vi "RxImgWithCLUT.vi"() -> ()   [LabVIEW 2016]
panel:
  out "Image Type":T1 items=["Grayscale (U8)", "Grayscale (I16)", "Grayscale (SGL)", "Complex (CSG)", "RGB (U32)", "HSL (U32)", "RGB (U64)", "Grayscale (U16)"]
  out "Image":T2(plugin-control)
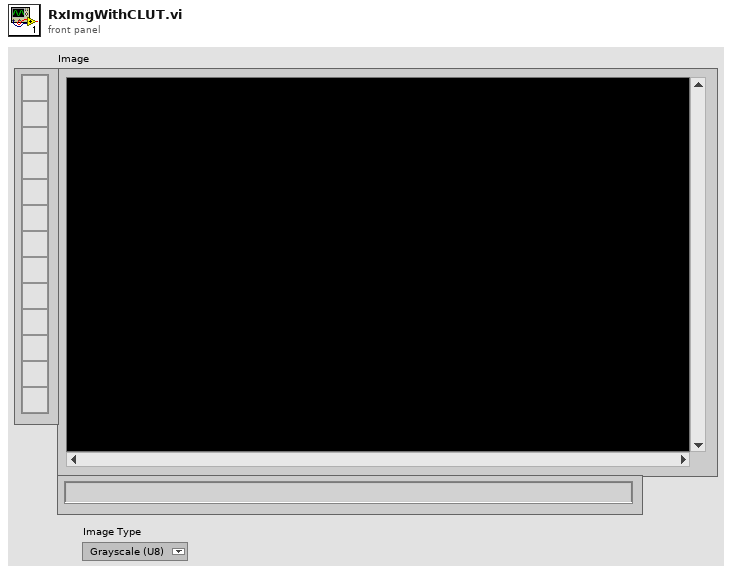
[diagram p1: front panel]
types:
  T1 = typedef "Image Type" = u32
  T2 = typedef "IMAQ Image.ctl" = refnum<image>
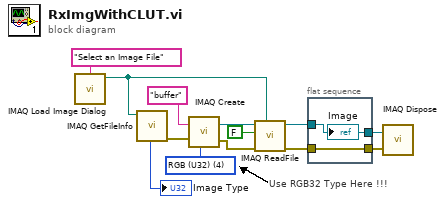
[diagram p0: block diagram]
diagram:
  w1 = T1 4 items=["Grayscale (U8)", "Grayscale (I16)", "Grayscale (SGL)", "Complex (CSG)", "RGB (U32)", "HSL (U32)", "RGB (U64)", "Grayscale (U16)"] ("Image Type")
  # "Use RGB32 Type Here !!!"
  n1 = call "IMAQ Load Image Dialog"("Prompt"="Select an Image File" ("prompt")) -> ("Path"=w5:path)  [unwired: 8 in, 2 out]
  n2 = call "IMAQ GetFileInfo"("File Path"=w5) -> ("error out"=w4:errorcluster, "Image Type"=→"Image Type":T1)  [unwired: 4 in, 5 out]
  n3 = call "IMAQ Create"("Image Name"="buffer", "Image Type"=w1, "error in (no error)"=w4) -> ("New Image"=w12:T2, "error out"=w11:errorcluster)  [unwired: 2 in]
  n4 = call "IMAQ ReadFile"("File Path"=w5, "error in (no error)"=w11, "Load Color Palette? (No)"=FALSE, "Image"=w12) -> ("error out"=w8:errorcluster, "Image Out"=w10:T2)  [unwired: 3 in, 3 out]
  n5 = flat-sequence {
    tunnel: w10 -> [w14]
    tunnel: [w15] -> w9
    tunnel: w8 -> [w15]
    tunnel: [w14] -> w7
    frame #0 {
      "Image" <- w14
    }
  }
  n6 = call "IMAQ Dispose"("Image"=w7, "error in (no error)"=w9) -> ()  [unwired: 4 in, 1 out]
